vi "HW_GEN - Search ParaValue According to ParaName.vi"(7 "element":string, 10 "Paravalues[]":string[](array[string]), 11 "ParaNames[]":string[](array[string])) -> (3 "value":string)   [LabVIEW 2016]
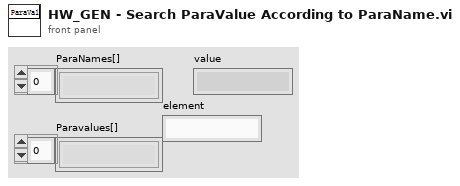
[diagram p1: front panel]
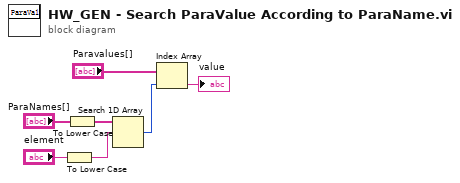
[diagram p0: block diagram]
diagram:
  n1 = To Lower Case(string="element") -> (all lower case string=w2:string)
  n2 = To Lower Case(string="ParaNames[]") -> (all lower case string=w1:string[])
  n3 = Search 1D Array(1D array=w1, element=w2) -> (index of element=w4:i32)  [unwired: 1 in]
  n4 = Index Array(array="Paravalues[]", index=w4) -> (element=→"value":string)
